vi "basic functionality test (multiple functions).vi"() -> ()   [LabVIEW 2020, in "mysql.lvlib" / "mysql.lvclass"]
uses:
  mysql.net/mysql.lvclass
panel:
  out "tables":string[](array[string])
  out "Database metadata":string[][](array[string])
  out "Columns out":string[](array[string])
  out "mysql out":refnum<class "mysql.lvclass">
  out "error out":errorcluster
  in  "Connection string":string="server=127.0.0.1;uid=root;pwd=Nitrog3n;database=test"
  in  "error in (no error)":errorcluster
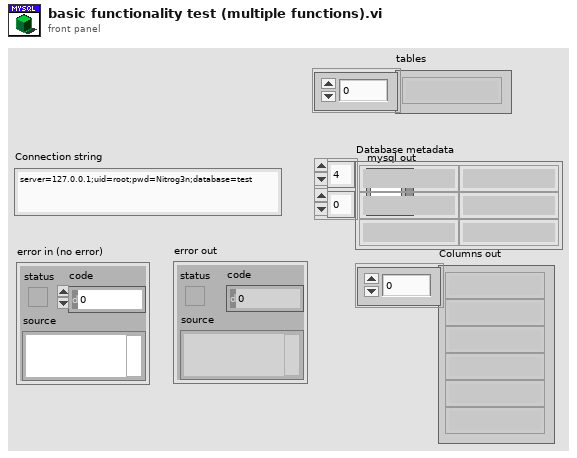
[diagram p1: front panel]
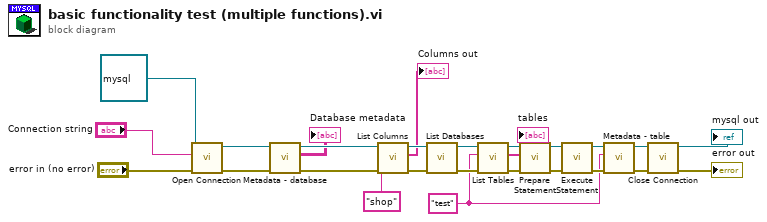
[diagram p0: block diagram]
diagram:
  w1 = "test" ("database")
  n1 = call-dynamic "Open Connection.vi"("error in (no error)"="error in (no error)", "Connection string"="Connection string", "mysql in"=refnum<class "mysql.lvclass"> refnum) -> ("error out"=w7:errorcluster, "mysql out"=w9:refnum<class "mysql.lvclass">)  [unwired: 7 in]
  n2 = call-dynamic "Metadata - database.vi"("error in (no error)"=w7, "mysql in"=w9) -> ("error out"=w6:errorcluster, "Database metadata"=→"Database metadata":string[][], "mysql out"=w8:refnum<class "mysql.lvclass">)  [unwired: 7 in]
  n3 = call-dynamic "List Columns.vi"("error in (no error)"=w6, "schema.table in"="shop" ("Table in"), "mysql in"=w8) -> ("error out"=w25:errorcluster, "Columns out"=→"Columns out":string[], "mysql out"=w26:refnum<class "mysql.lvclass">)  [unwired: 5 in, 1 out]
  n4 = call-dynamic "List Databases.vi"("error in (no error)"=w25, "mysql in"=w26) -> ("error out"=w23:errorcluster, "mysql out"=w24:refnum<class "mysql.lvclass">)  [unwired: 7 in, 1 out]
  n5 = call-dynamic "List Tables.vi"("error in (no error)"=w23, "database"=w1, "mysql in"=w24) -> ("error out"=w21:errorcluster, "tables"=→"tables":string[], "mysql out"=w22:refnum<class "mysql.lvclass">)  [unwired: 6 in]
  n6 = call-dynamic "Prepare Statement.vi"("error in (no error)"=w21, "mysql in"=w22) -> ("error out"=w19:errorcluster, "mysql out"=w20:refnum<class "mysql.lvclass">)  [unwired: 7 in, 1 out]
  n7 = call-dynamic "Execute Statement.vi"("error in (no error)"=w19, "mysql in"=w20) -> ("error out"=w17:errorcluster, "mysql out"=w18:refnum<class "mysql.lvclass">)  [unwired: 7 in, 1 out]
  n8 = call-dynamic "Metadata - table.vi"("error in (no error)"=w17, "Database in"=w1, "mysql in"=w18) -> ("error out"=w4:errorcluster, "mysql out"=w3:refnum<class "mysql.lvclass">)  [unwired: 6 in, 1 out]
  n9 = call-dynamic "Close Connection.vi"("error in (no error)"=w4, "mysql in"=w3) -> ("error out"=→"error out":errorcluster, "mysql out"=→"mysql out":refnum<class "mysql.lvclass">)  [unwired: 8 in]
